vi "MMI_PAS_StrDismantle.vi"(1 "LogEvent":refnum<vi>, 2 "VCI_CAN_OBJ_R":T1) -> (0 "MMI_PAS_CmdCluster":T2 {"iBooster制动模式" items=["NoRequest", "ComfortMode", "SportMode ", "预留"]; "EVA与驾驶模式联动" items=["无联动", "联动", "预留"]; "EVA排气声浪开关" items=["无响应", "开", "关", "预留"]; "SUM与驾驶模式联动选择" items=["无联动", "联动", "预留"]; "SUM模式选择" items=["No Action", "Confort", "Sport", "预留"]; "泊入功能选择" items=["无按键按下", "水平按下", "垂直按下", "预留"]; "PAS-APA功能确认或关闭" items=["无按键按下", "确认键按下", "终止键按下", "预留"]; "泊入泊出功能选择" items=["未按下", "PSC按下", "POC按下", "预留"]; "环视摄像头功能状态" items=["未激活", "激活", "保持", "失败"]; "导航状态" items=["正常", "失败", "预留"]; "当前所处道路类型" items=["未知", "高速路", "乡道", "国道", "省道", "主干道", "分叉路", "其它"]; "来自地图数据库的限速" scale=0.0..255.0; "前方匝道距离" items=["无匝道", "1000m", "500m", "200m", "预留"]})   [LabVIEW 2013]
uses:
  Log.ctl
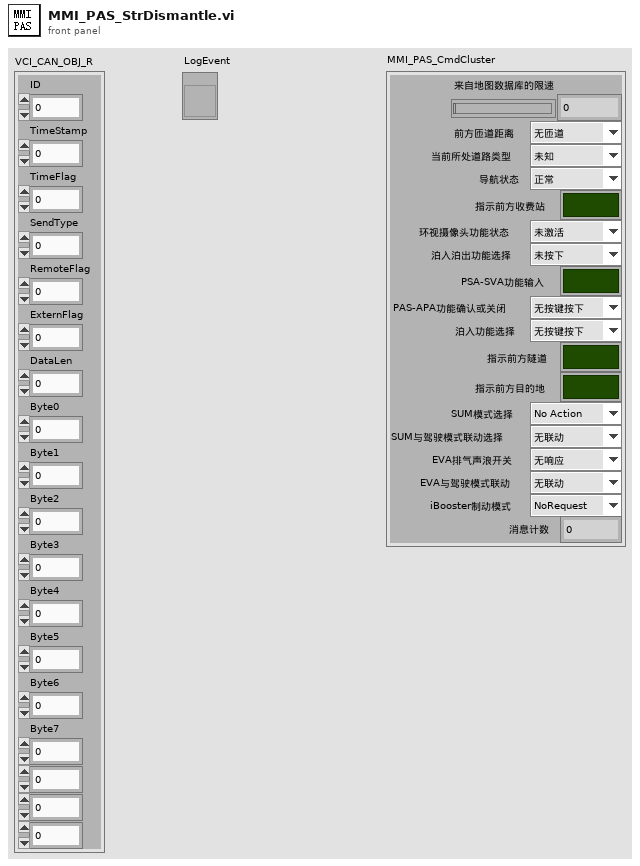
[diagram p1: front panel]
types:
  T1 = cluster{"ID":u32, "TimeStamp":u32, "TimeFlag":u8, "SendType":u8, "RemoteFlag":u8, "ExternFlag":u8, "DataLen":u8, "Byte0":u8, "Byte1":u8, "Byte2":u8, "Byte3":u8, "Byte4":u8, "Byte5":u8, "Byte6":u8, "Byte7":u8, u8, u8, u8}
  T2 = cluster{"来自地图数据库的限速":i32, " 前方匝道距离":u16, "当前所处道路类型":u16, "导航状态":u16, "指示前方收费站":bool, "环视摄像头功能状态":u16, "泊入泊出功能选择":u16, "PSA-SVA功能输入":bool, "PAS-APA功能确认或关闭":u16, "泊入功能选择":u16, "指示前方隧道":bool, "指示前方目的地":bool, "SUM模式选择":u16, "SUM与驾驶模式联动选择":u16, "EVA排气声浪开关":u16, "EVA与驾驶模式联动":u16, "iBooster制动模式":u16, "消息计数":u8}
  T3 = typedef "Log.ctl" = cluster{"Event":string, "Value":variant}
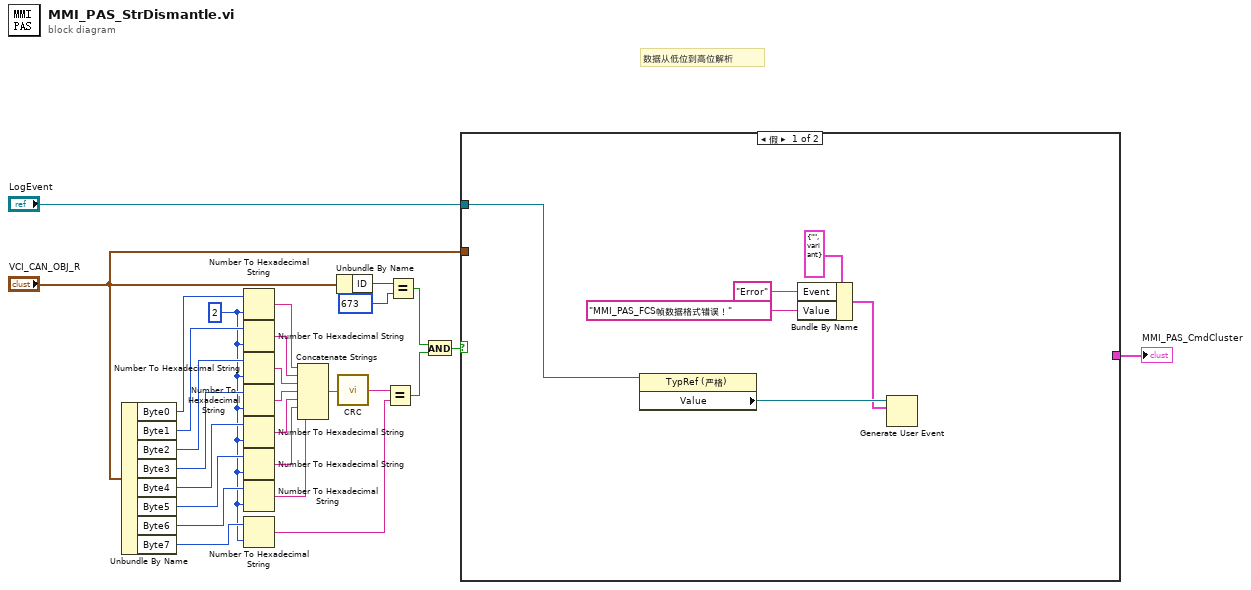
[diagram p0: block diagram]
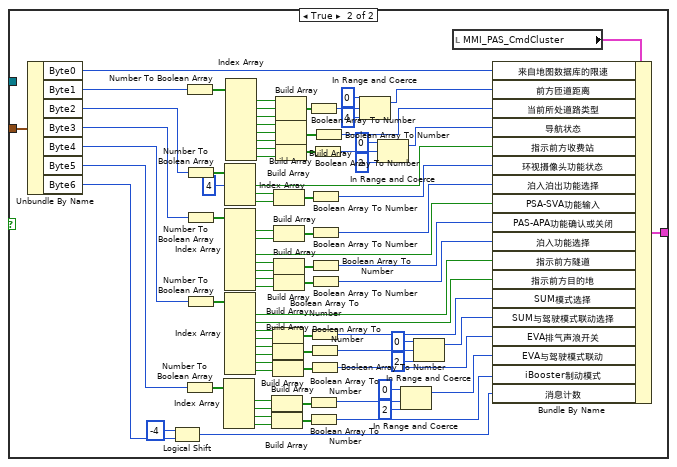
[diagram p2: hidden frame]
diagram:
  w8 = 2
  # "数据从低位到高位解析"
  n1 = Unbundle By Name("VCI_CAN_OBJ_R") -> ("Byte0"=w24:u8, "Byte1"=w23:u8, "Byte2"=w22:u8, "Byte3"=w21:u8, "Byte4"=w20:u8, "Byte5"=w19:u8, "Byte6"=w18:u8, "Byte7"=w9:u8)
  n2 = Number To Hexadecimal String(1:w8, 2:w24) -> (0:w17:string)
  n3 = Number To Hexadecimal String(1:w8, 2:w23) -> (0:w16:string)
  n4 = Number To Hexadecimal String(1:w8, 2:w22) -> (0:w15:string)
  n5 = Number To Hexadecimal String(1:w8, 2:w21) -> (0:w14:string)
  n6 = Number To Hexadecimal String(1:w8, 2:w20) -> (0:w13:string)
  n7 = Number To Hexadecimal String(1:w8, 2:w19) -> (0:w12:string)
  n8 = Number To Hexadecimal String(1:w8, 2:w18) -> (0:w11:string)
  n9 = Number To Hexadecimal String(1:w8, 2:w9) -> (0:w6:string)
  n10 = Concatenate Strings(w17, w16, w15, w14, w13, w12, w11) -> (w10:string)
  n11 = Unbundle By Name("VCI_CAN_OBJ_R") -> ("ID"=w26:u32)
  n12 = call "CRC.vi"("StrIn"=w10) -> ("StrOut"=w7:string)
  n13 = Equal?(x=w7, y=w6) -> (x = y?=w4:bool)
  n14 = Equal?(x=w26, y=u16 673) -> (x = y?=w3:bool)
  n15 = And(x=w3, y=w4) -> (x .and. y?=w5:bool)
  n16 = case shown="假" w5 {
    tunnel: [_ w88] -> w27
    tunnel: "VCI_CAN_OBJ_R" -> [_ w43]
    tunnel: "LogEvent" -> [w29 _]
    frame False {
      n17 = property class="TypRef (严格)"(reference=w29) -> ("Value"=w33:refnum<user-event>)  [unwired: 1 in, 2 out]
      n18 = Bundle By Name(cluster=T3 {"Event"="", "Value"=variant} ("Log"), "Event"="Error", "Value"="MMI_PAS_FCS帧数据格式错误！" ("消息")) -> (w30:T3)
      n19 = Generate User Event(user event=w33, event data cluster=w30) -> ()  [unwired: 2 in, 2 out]
    }
    frame True {
      n20 = Unbundle By Name(w43) -> ("Byte0"=w42:u8, "Byte1"=w41:u8, "Byte2"=w40:u8, "Byte3"=w39:u8, "Byte4"=w38:u8, "Byte5"=w37:u8, "Byte6"=w36:u8)
      n21 = Logical Shift(y=i16 -4, x=w36) -> (x << y=w35:u8)
      n22 = Number To Boolean Array(number=w41) -> (Boolean array=w115:bool[])
      n23 = Number To Boolean Array(number=w37) -> (Boolean array=w55:bool[])
      n24 = Number To Boolean Array(number=w40) -> (Boolean array=w95:bool[])
      n25 = Number To Boolean Array(number=w39) -> (Boolean array=w87:bool[])
      n26 = Number To Boolean Array(number=w38) -> (Boolean array=w73:bool[])
      n27 = Index Array(array=w55) -> (element #1=w52:bool, element #2=w50:bool, element #3=w51:bool, element #4=w49:bool)  [unwired: 4 in]
      n28 = Index Array(array=w95, index #1=4 ("索引")) -> (element #1=w93:bool, element #2=w92:bool, element #3=w91:bool)  [unwired: 2 in]
      n29 = Index Array(array=w87) -> (element #1=w84:bool, element #2=w85:bool, element #4=w82:bool, element #5=w80:bool, element #6=w79:bool, element #7=w76:bool, element #8=w75:bool)  [unwired: 8 in, 1 out]
      n30 = Index Array(array=w73) -> (element #1=w72:bool, element #2=w71:bool, element #3=w68:bool, element #4=w67:bool, element #5=w66:bool, element #6=w65:bool, element #7=w64:bool, element #8=w63:bool)  [unwired: 8 in]
      n31 = Index Array(array=w115) -> (element #1=w114:bool, element #2=w113:bool, element #3=w112:bool, element #4=w106:bool, element #5=w105:bool, element #6=w104:bool, element #7=w101:bool, element #8=w100:bool)  [unwired: 8 in]
      n32 = Build Array(w52, w50) -> (w53:bool[])
      n33 = Build Array(w51, w49) -> (w54:bool[])
      n34 = Build Array(w68, w67) -> (w69:bool[])
      n35 = Build Array(w66, w65) -> (w70:bool[])
      n36 = Build Array(w64, w63) -> (w62:bool[])
      n37 = Build Array(w92, w91) -> (w90:bool[])
      n38 = Build Array(w84, w85) -> (w86:bool[])
      n39 = Build Array(w80, w79) -> (w81:bool[])
      n40 = Build Array(w76, w75) -> (w77:bool[])
      n41 = Build Array(w114, w113, w112) -> (w111:bool[])
      n42 = Build Array(w106, w105, w104) -> (w102:bool[])
      n43 = Build Array(w101, w100) -> ()  [unwired: 1 out]
      n44 = Boolean Array To Number(Boolean array=w111) -> (number=w110:u32)
      n45 = Boolean Array To Number(Boolean array=w53) -> (number=w48:u32)
      n46 = Boolean Array To Number(Boolean array=w54) -> (number=w44:u32)
      n47 = Boolean Array To Number(Boolean array=w69) -> (number=w61:u32)
      n48 = Boolean Array To Number(Boolean array=w70) -> (number=w57:u32)
      n49 = Boolean Array To Number(Boolean array=w62) -> (number=w56:u32)
      n50 = Boolean Array To Number(Boolean array=w90) -> (number=w89:u32)
      n51 = Boolean Array To Number(Boolean array=w86) -> (number=w83:u32)
      n52 = Boolean Array To Number(Boolean array=w81) -> (number=w78:u32)
      n53 = Boolean Array To Number(Boolean array=w77) -> (number=w74:u32)
      n54 = Boolean Array To Number(Boolean array=w102) -> (number=w99:u32)
      n55 = Boolean Array To Number(Boolean array=w102) -> (number=w103:u32)
      n56 = In Range and Coerce(upper limit=u32 0 ("上限"), x=w110, lower limit=u32 4 ("下限")) -> (coerced(x)=w107:u32)  [unwired: 1 out]
      n57 = In Range and Coerce(upper limit=u32 0 ("上限"), x=w99, lower limit=u32 2 ("下限")) -> (coerced(x)=w96:u32)  [unwired: 1 out]
      n58 = In Range and Coerce(upper limit=u32 0 ("上限"), x=w48, lower limit=u32 2 ("下限")) -> (coerced(x)=w45:u32)  [unwired: 1 out]
      n59 = In Range and Coerce(upper limit=u32 0 ("上限"), x=w57, lower limit=u32 2 ("下限")) -> (coerced(x)=w58:u32)  [unwired: 1 out]
      n60 = local read "MMI_PAS_CmdCluster"() -> (w116:T2)
      n61 = Bundle By Name(cluster=w116, "来自地图数据库的限速"=w42, "前方匝道距离"=w107, "当前所处道路类型"=w103, "导航状态"=w96, "指示前方收费站"=w93, "环视摄像头功能状态"=w89, "泊入泊出功能选择"=w83, "PSA-SVA功能输入"=w82, "PAS-APA功能确认或关闭"=w78, "泊入功能选择"=w74, "指示前方隧道"=w72, "指示前方目的地"=w71, "SUM模式选择"=w61, "SUM与驾驶模式联动选择"=w58, "EVA排气声浪开关"=w56, "EVA与驾驶模式联动"=w45, "iBooster制动模式"=w44, "消息计数"=w35) -> (w88:T2)
    }
  }
  "MMI_PAS_CmdCluster" <- w27
